vi "DecimalToCommand.vi"(2 "Decimal":u16) -> (5 "HiByte":u8, 6 "LoByte":u8)   [LabVIEW 2017, in "Spectral Products CM110.lvlib"]
uses:
  Spectral Products CM110.lvlib
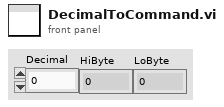
[diagram p1: front panel]
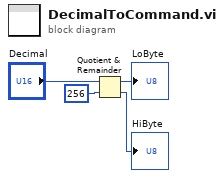
[diagram p0: block diagram]
diagram:
  n1 = Quotient & Remainder(x="Decimal", y=256) -> (x-y*floor(x/y)=→"LoByte":i32, floor(x/y)=→"HiByte":i32)
